vi "rad2deg.vi"(2 "deg":dbl, 3 "rad":dbl) -> (0 "rad":dbl, 1 "deg":dbl)   [LabVIEW 2011]
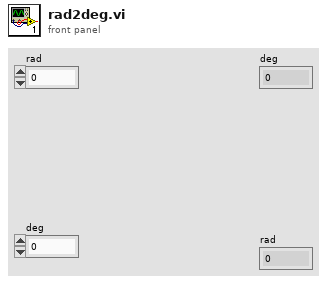
[diagram p1: front panel]
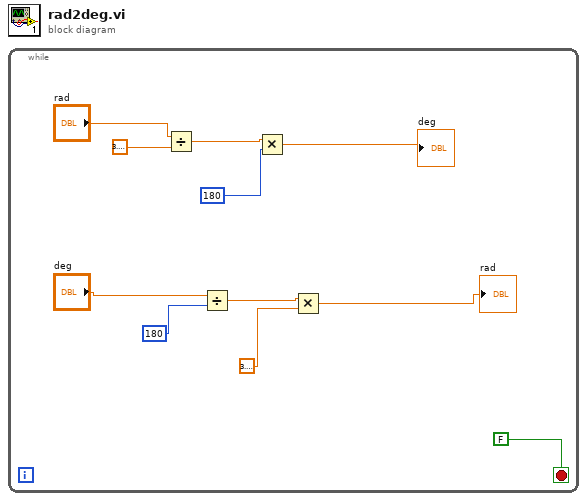
[diagram p0: block diagram]
diagram:
  n1 = while {
    stop <- FALSE stop-if-true
    n2 = Divide(x="rad", y=3.141592653589793) -> (x/y=w9:dbl)
    n3 = Divide(x="deg", y=180) -> (x/y=w6:dbl)
    n4 = Multiply(x=w9, y=180) -> (x*y=→"deg":dbl)
    n5 = Multiply(x=w6, y=3.141592653589793) -> (x*y=→"rad":dbl)
  }
